vi "Print HTML Report ext.vi"(0 "report in":T1, 9 "IE Print Options":i32(ring)=1 items=["OLECMDEXECOPT_DODEFAULT", "OLECMDEXECOPT_PROMPTUSER", "OLECMDEXECOPT_DONTPROMPTUSER", "OLECMDEXECOPT_SHOWHELP"], 11 "error in (no error)":errorcluster) -> (4 "report out":T1, 15 "error out":errorcluster)   [LabVIEW 2017]
doc: "This VI prints an HTML Report using Internet Explorer.\n\nextended to allow option of displaying IE print dialog."
uses:
  <vilib>/Utility/NIReport.llb/Generate Report Object Reference.ctl
  <vilib>/Utility/NIReport.llb/NI_report.lvclass
  <vilib>/printing/ReportDocExtensions.llb/File_types_for_reports.ctl
  <vilib>/registry/registry.llb/Registry RtKey.ctl
  <vilib>/registry/registry.llb/Read Registry Value Simple STR.vi
  <vilib>/Utility/NIReport.llb/NI_ReportGenerationCore.lvlib
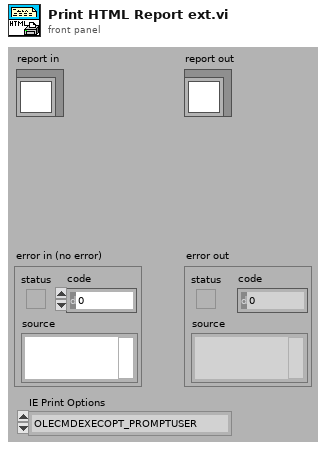
[diagram p1: front panel]
types:
  T1 = typedef "Generate Report Object Reference.ctl" = refnum<class "NI_report.lvclass">
  T2 = typedef "Registry RtKey.ctl" = enum32{"HKEY_CLASSES_ROOT", "HKEY_CURRENT_USER", "HKEY_LOCAL_MACHINE", "HKEY_USERS", "HKEY_PERFORMANCE_DATA", "HKEY_CURRENT_CONFIG", "HKEY_DYN_DATA"}
  T3 = enum32{"KEY_QUERY_VALUE", "KEY_SET_VALUE", "KEY_CREATE_SUB_KEY", "KEY_ENUMERATE_SUB_KEYS", "KEY_NOTIFY", "KEY_CREATE_LINK", "KEY_READ", "KEY_WRITE", "KEY_ALL_ACCESS", "KEY_READ | KEY_WRITE"}
  T4 = typedef "NI_ReportGenerationCore.lvlib/File_types_for_reports.ctl" = enum16{".jpg", ".png", ".html", ".gif"}
  T5 = typedef "Registry refnum.ctl" = refnum<k1>
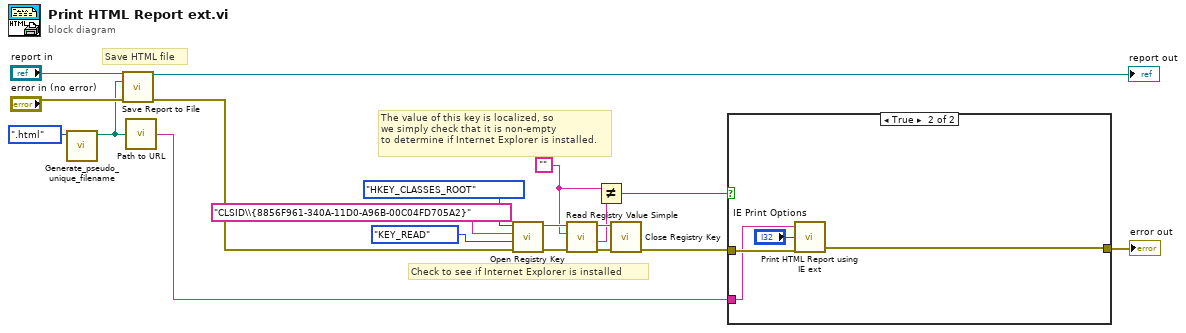
[diagram p0: block diagram]
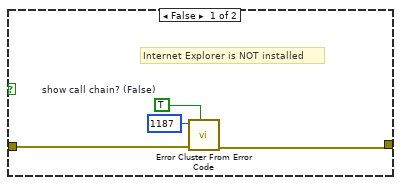
[diagram p2: hidden frame]
diagram:
  w1 = ""
  # "The value of this key is localized, so\nwe simply check that it is non-empty\nto determine if Internet Explorer is installed."
  # "Check to see if Internet Explorer is installed"
  # "Save HTML file"
  n1 = call <vilib>:"Generate_pseudo_unique_filename.vi"("file type(.jpg)"=File_types_for_reports.".html") -> ("generated path"=w15:path)  [unwired: 8 in, 2 out]
  n2 = call-dynamic "Save Report to File.vi"("report in"="report in", "report file path"=w15, "error in (no error)"="error in (no error)") -> ("report out"=→"report out":T1, "error out"=w3:errorcluster)  [unwired: 11 in]
  n3 = call <vilib>:"Path to URL.vi"("path"=w15) -> ("url"=w14:string)
  n4 = call <vilib>:"Open Registry Key.vi"("error in (no error)"=w3, "security access mask (KEY_READ | KEY_WRITE)"=T3."KEY_READ", "subkey"="CLSID\\{8856F961-340A-11D0-A96B-00C04FD705A2}", "root key (HKEY_LOCAL_MACHINE)"=Registry_RtKey."HKEY_CLASSES_ROOT") -> ("error out"=w9:errorcluster, "refnum out"=w7:T5)  [unwired: 6 in]
  n5 = call-poly <vilib>:"Read Registry Value Simple.vi"("error in (no error)"=w9, "value"=w1, "refnum"=w7) -> ("error out"=w6:errorcluster, "String/Binary data"=w12:string, "refnum out"=w13:T5)  [unwired: 3 in, 1 out]
  n6 = Not Equal?(x=w1, y=w12) -> (x != y?=w5:bool)
  n7 = call <vilib>:"Close Registry Key.vi"("error in (no error)"=w6, "refnum"=w13) -> ()  [unwired: 5 in, 1 out]
  n8 = case shown="True" w5 {
    tunnel: [w20 w24] -> w2
    tunnel: w6 -> [w21 w26]
    tunnel: w14 -> [_ w25]
    frame False {
      w19 = TRUE  # show call chain? (False)
      # "Internet Explorer is NOT installed"
      n9 = call <vilib>:"Error Cluster From Error Code.vi"("show call chain? (False)"=w19, "error in (no error)"=w21, "error code (0)"=1187) -> ("error out"=w20:errorcluster)  [unwired: 6 in]
    }
    frame True {
      n10 = call "Print HTML Report using IE ext.vi"("Error In"=w26, "IE Print Options"="IE Print Options", "Path to HTML"=w25) -> ("Error Out"=w24:errorcluster)  [unwired: 2 in]
    }
  }
  "error out" <- w2
